vi "Create_Eval_Tmp.vi"   [LabVIEW 2016]
uses:
  Evaluation Interface/SeqAuto IEvaluation.lvlibp/TestStand API Tools/Evaluation Actions/Includes/Controls/TSAT Eval SI Unit Scaling.ctl
  Evaluation Interface/SeqAuto IEvaluation.lvlibp/TestStand API Tools/Evaluation Actions/Includes/Controls/TSAT Evaluation.ctl
  LTE_ACP.lvclass
types:
  T1 = typedef "SeqAuto IEvaluation.lvlibp/TestStand API Tools (TSAT).lvlib/TSAT Evaluation Actions.lvlib/TSAT Eval SI Unit Scaling.ctl" = i16
  T2 = typedef "SeqAuto IEvaluation.lvlibp/TestStand API Tools (TSAT).lvlib/TSAT Evaluation Actions.lvlib/TSAT Evaluation.ctl" = cluster{"Test Name":string, "Pin":string, "Units":string, "SI Scaling":T1, "Test Number":i32, "Published Data Id":string, "Low Limit":dbl, "High Limit":dbl, "Export Data Location":string, "Fail Bin":i64}
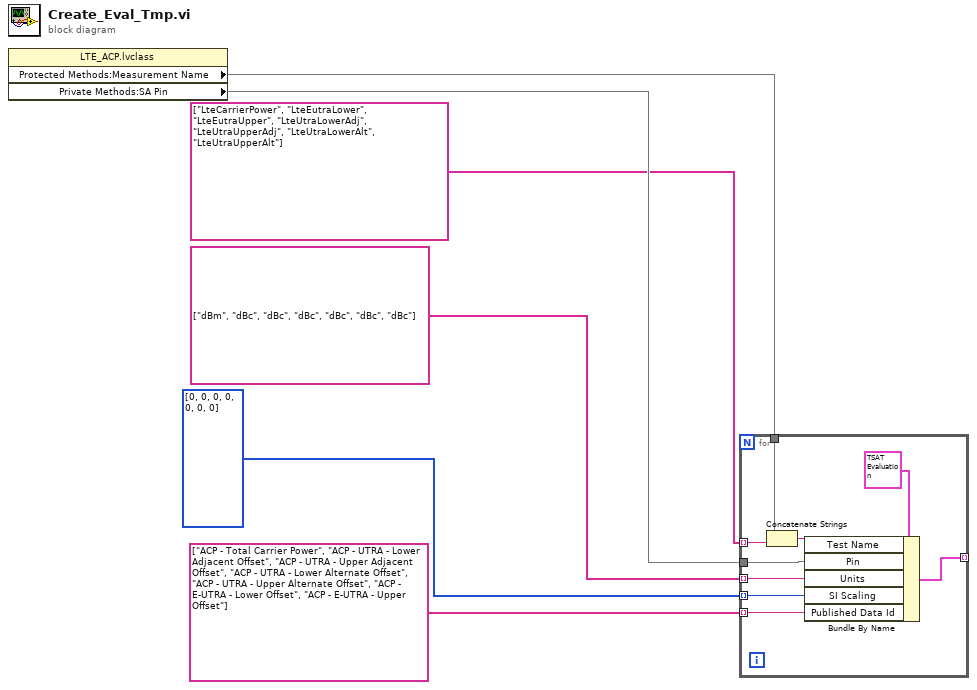
[diagram p0: block diagram]
diagram:
  w5 = T1[] [0, 0, 0, 0, 0, 0, 0] items=["femto"=-15, "pico"=-12, "nano"=-9, "micro"=-6, "milli"=-3, "percent"=-2, ""=0, "kilo"=3, "mega"=6, "giga"=9, "tera"=12]
  n1 = property class="LTE_ACP.lvclass"() -> (reference out=w7:refnum<class "LTE_ACP.lvclass">, error in=w9:errorcluster, error out=w8:errorcluster, "Protected Methods:Measurement Name"=w1, "Private Methods:SA Pin"=w3)  [unwired: 1 in]
  n2 = for {
    tunnel: [w17] -> _ mode=indexing
    tunnel: string[] ["ACP - Total Carrier Power", "ACP - UTRA - Lower Adjacent Offset", "ACP - UTRA - Upper Adjacent Offset", "ACP - UTRA - Lower Alternate Offset", "ACP - UTRA - Upper Alternate Offset", "ACP - E-UTRA - Lower Offset", "ACP - E-UTRA - Upper Offset"] ("Array") -> [w16] mode=indexing
    tunnel: w5 -> [w15] mode=indexing
    tunnel: string[] ["dBm", "dBc", "dBc", "dBc", "dBc", "dBc", "dBc"] ("Array") -> [w14] mode=indexing
    tunnel: w3 -> [w13]
    tunnel: string[] ["LteCarrierPower", "LteEutraLower", "LteEutraUpper", "LteUtraLowerAdj", "LteUtraUpperAdj", "LteUtraLowerAlt", "LteUtraUpperAlt"] -> [w12] mode=indexing
    tunnel: w1 -> [w10]
    n3 = Concatenate Strings(w10, w12) -> (w11:string)
    n4 = Bundle By Name(cluster=T2 {"Test Name"="", "Pin"="", "Units"="", "SI Scaling"=0, "Test Number"=0, "Published Data Id"="", "Low Limit"=-999999.0, "High Limit"=999999.0, "Export Data Location"="", "Fail Bin"=-1} ("Evaluation"), "Test Name"=w11, "Pin"=w13, "Units"=w14, "SI Scaling"=w15, "Published Data Id"=w16) -> (w17:T2)
  }
